vi "Check for Server.vi"(8 "error in (no error)":errorcluster) -> (0 "error out":errorcluster, 1 "WLM server running?":bool, 2 "return value":i32)   [LabVIEW 2017, in "HighFinesse WS5.lvlib"]
doc: "Checks to see if one or more instances of the wavelength meter server are running."
uses:
  HighFinesse WS5.lvlib
  wlmData.dll
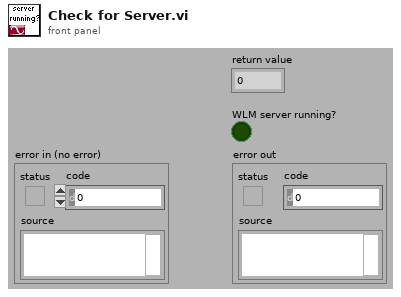
[diagram p1: front panel]
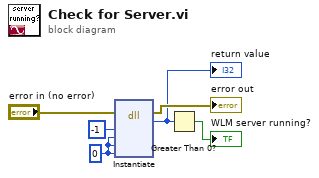
[diagram p0: block diagram]
diagram:
  w4 = 0 ("P2")
  n1 = dll-call lib="C:/LabVIEW-programs/Instruments/Wavelength meter/HighFinesse WS5/wlmData.dll" fn="Instantiate"(error in="error in (no error)", "RFC"=-1, "Mode"=w4, "P1"=w4, "P2"=w4) -> (error out=→"error out":errorcluster, "return type"=w2:i32)  [unwired: 6 in, 1 out]
  "return value" <- w2
  n2 = Greater Than 0?(x=w2) -> (x > 0?=→"WLM server running?":bool)
